vi "Self Event Alias.vi"(11 "Template Event in":refnum<class "Template Event.lvclass">) -> (2 "Self Event Alias":string)   [LabVIEW 2021, in "_Template.lvlib" / "Templates.lvlib" / "Template Event.lvlib" / "Template Event.lvclass"]
uses:
  Template Event.lvclass
  Template Event.lvclass/Template Event.ctl
  <vilib>/jettl/jettl/jettl/Event/Event.lvclass
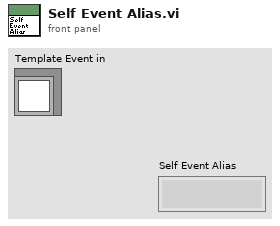
[diagram p1: front panel]
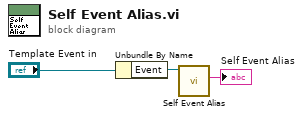
[diagram p0: block diagram]
diagram:
  n1 = Unbundle By Name("Template Event in") -> ("Event"=w2:refnum<class "Event.lvclass">)
  n2 = call-dynamic "Self Event Alias.vi"("Event in"=w2) -> ("Self Event Alias"=→"Self Event Alias":string)  [unwired: 10 in]
